vi "Stream_Close.vi"(8 "error in (no error)":errorcluster, 11 "Stream":refnum<k24>) -> (0 "error out":errorcluster)   [LabVIEW 2018, in "HttpClient_NET.lvlib" / "HttpContent.lvclass"]
uses:
  HttpContent.lvclass
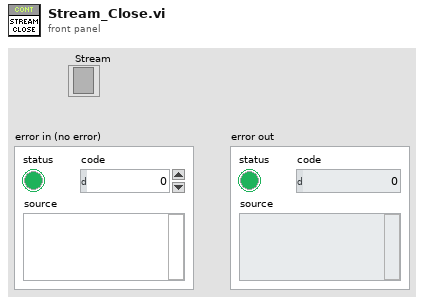
[diagram p1: front panel]
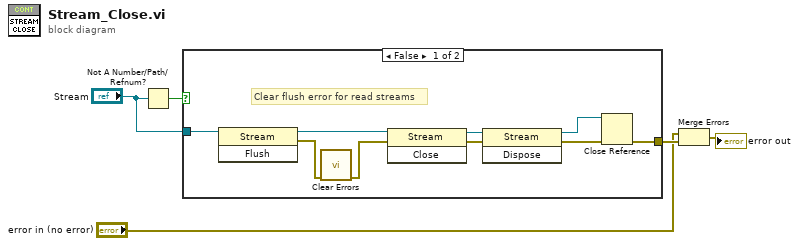
[diagram p0: block diagram]
diagram:
  n1 = Not A Number/Path/Refnum?(number/path/refnum="Stream") -> (NaN/Path/Refnum?=w3:bool)
  n2 = case shown="False" w3 {
    tunnel: [w14 _] -> w5
    tunnel: "Stream" -> [w8 _]
    frame False {
      # "Clear flush error for read streams"
      n3 = invoke class="Stream" method="Flush"(reference=w8) -> (reference out=w9:refnum<k24>, error out=w7:errorcluster)  [unwired: 2 in, 1 out]
      n4 = call <vilib>:"Clear Errors.vi"("error in (no error)"=w7) -> ("error out"=w6:errorcluster)  [unwired: 5 in, 1 out]
      n5 = invoke class="Stream" method="Close"(reference=w9, error in=w6) -> (reference out=w10:refnum<k24>, error out=w11:errorcluster)  [unwired: 1 in, 1 out]
      n6 = invoke class="Stream" method="Dispose"(reference=w10, error in=w11) -> (reference out=w13:refnum<k24>, error out=w12:errorcluster)  [unwired: 1 in, 1 out]
      n7 = Close Reference(reference=w13, error in (no error)=w12) -> (error out=w14:errorcluster)
    }
    frame True {
    }
  }
  n8 = Merge Errors("error in (no error)", w5) -> (→"error out":errorcluster)
